vi "StrToChrArray.vi"(1 "String in":string) -> (0 "Array char":string[](array[string]))   [LabVIEW 2010]
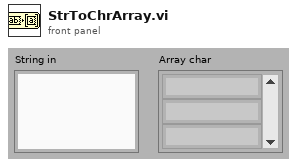
[diagram p1: front panel]
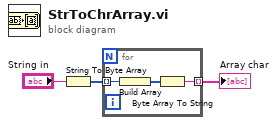
[diagram p0: block diagram]
diagram:
  n1 = String To Byte Array(string="String in") -> (unsigned byte array=w2:u8[])
  n2 = for {
    tunnel: w2 -> [w6] mode=indexing
    tunnel: [w4] -> w1 mode=indexing
    n3 = Build Array(w6) -> (w5:u8[])
    n4 = Byte Array To String(unsigned byte array=w5) -> (string=w4:string)
  }
  "Array char" <- w1
